vi "Calculation for full mode.vi"(0 "Опускания подложки до раствора":dbl[](array[numeric])=[2.9, 2.9, 2.9, 2.9], 1 "Опускания подложки в растворе":dbl[](array[numeric])=[1.0, 1.0, 1.0, 1.0], 2 "Подъема подложки из раствора":dbl[](array[numeric])=[1.0, 1.0, 1.0, 1.0], 3 "Подъема подложки над раствором":dbl[](array[numeric])=[2.9, 2.9, 2.9, 2.9], 4 "Steps for full mode":dbl, 6 "Текущий раствор":i32, 8 "Нахождения в растворе":dbl[](array[numeric])=[1.0, 1.0, 1.0, 1.0] caption="Время нахождения в растворе (секунды)", 10 "Задержки после подъема из раствора":dbl[](array[numeric])=[0.0, 0.0, 0.0, 0.0]) -> (11 "Время задержки после подъема":dbl, 13 "Время нахождения в растворе":dbl, 14 "Скорость 4":dbl, 15 "Скорость 3":dbl, 16 "Скорость 2":dbl, 17 "Скорость 1":dbl, 18 "Кол-во шагов 1":dbl)   [LabVIEW 2016]
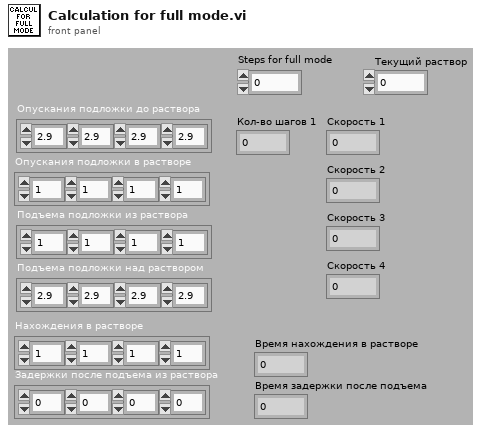
[diagram p1: front panel]
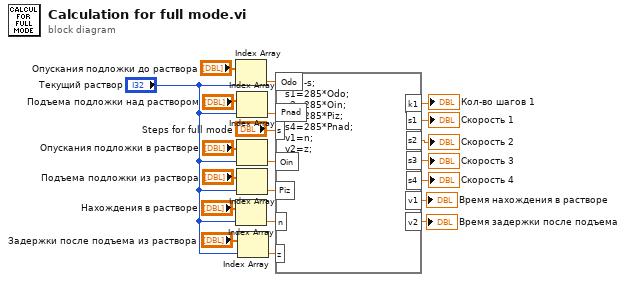
[diagram p0: block diagram]
diagram:
  n1 = Index Array(array="Опускания подложки до раствора", index="Текущий раствор") -> (element=w14:dbl)
  n2 = Index Array(array="Нахождения в растворе", index="Текущий раствор") -> (element=w6:dbl)
  n3 = Index Array(array="Подъема подложки над раствором", index="Текущий раствор") -> (element=w13:dbl)
  n4 = Index Array(array="Опускания подложки в растворе", index="Текущий раствор") -> (element=w10:dbl)
  n5 = Index Array(array="Подъема подложки из раствора", index="Текущий раствор") -> (element=w9:dbl)
  n6 = Index Array(array="Задержки после подъема из раствора", index="Текущий раствор") -> (element=w7:dbl)
  n7 = formula code="k1=-s;\ns1=285*Odo;\ns2=285*Oin;\ns3=285*Piz;\ns4=285*Pnad;\nv1=n;\nv2=z;"("Odo"=w14, "Pnad"=w13, "s"="Steps for full mode", "Oin"=w10, "Piz"=w9, "n"=w6, "z"=w7) -> ("k1"=→"Кол-во шагов 1":dbl, "s1"=→"Скорость 1":dbl, "s2"=→"Скорость 2":dbl, "s3"=→"Скорость 3":dbl, "s4"=→"Скорость 4":dbl, "v1"=→"Время нахождения в растворе":dbl, "v2"=→"Время задержки после подъема":dbl)
